vi "Write Image.vi"(0 "Session In":T1, 1 "Folder":string, 2 "Image Name":string, 3 "Camera Missing?":bool, 5 "Error In":errorcluster, 6 "Student ID":i32) -> (14 "Session Out":T1, 16 "Image Out":T2, 19 "Error Out":errorcluster)   [LabVIEW 2013]
uses:
  <vilib>/vision/Image Controls.llb/IMAQ Image.ctl
  <vilib>/userdefined/High Color/IMAQdx.ctl
  <vilib>/vision/driver/NI_Vision_Acquisition_Software.lvlib
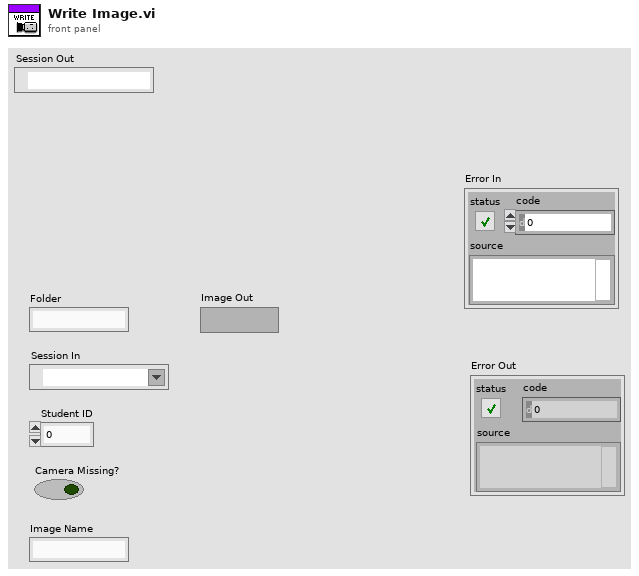
[diagram p1: front panel]
types:
  T1 = typedef "IMAQdx.ctl" = refnum<k21>
  T2 = typedef "IMAQ Image.ctl" = refnum<image>
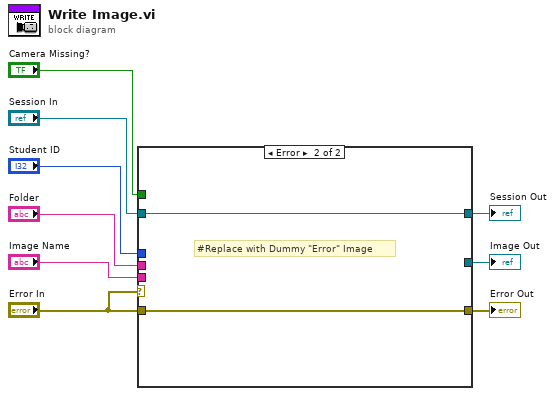
[diagram p0: block diagram]
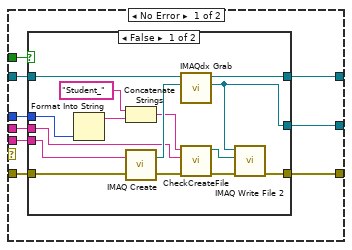
[diagram p2: hidden frame]
diagram:
  n1 = case shown="Error" "Error In" {
    tunnel: "Image Name" -> [w18 _]
    tunnel: "Folder" -> [w17 _]
    tunnel: "Student ID" -> [w16 _]
    tunnel: "Camera Missing?" -> [w15 _]
    tunnel: [w14 _] -> w5
    tunnel: "Session In" -> [w13 w36]
    tunnel: [w12 w36] -> w3
    tunnel: [w11 w37] -> w2
    tunnel: "Error In" -> [w10 w37]
    frame No Error {
      n2 = case shown="False" w15 {
        tunnel: w13 -> [w33 w35]
        tunnel: [w31 _] -> w14
        tunnel: w16 -> [w26 _]
        tunnel: w17 -> [w25 _]
        tunnel: w18 -> [w24 _]
        tunnel: [w23 w35] -> w12
        tunnel: [w21 w34] -> w11
        tunnel: w10 -> [w20 w34]
        frame False {
          n3 = Format Into String(w26) -> (resulting string=w28:string)  [unwired: 3 in, 1 out]
          n4 = Concatenate Strings("Student_" ("string"), w28) -> (w27:string)
          n5 = call "IMAQ Create"("Image Name"=w24, "error in (no error)"=w20) -> ("New Image"=w32:T2, "error out"=w19:errorcluster)  [unwired: 2 in, 1 out]
          n6 = call <vilib>:"IMAQdx Grab.vi"("Image In"=w32, "Session In"=w33) -> ("Image Out"=w31:T2, "Session Out"=w23:T1)  [unwired: 2 in, 6 out]
          n7 = call "CheckCreateFile.vi"("Error In"=w19, "Folder"=w25, "Image Name"=w27) -> ("Error Out"=w22:errorcluster, "File Path"=w30:path)  [unwired: 7 in]
          n8 = call-poly "IMAQ Write File 2"("error in (no error)"=w22, "File Path"=w30, "Image"=w31) -> ("error out"=w21:errorcluster)  [unwired: 7 in, 1 out]
        }
        frame True {
        }
      }
    }
    frame Error {
      # "#Replace with Dummy \"Error\" Image"
    }
  }
  "Image Out" <- w5
  "Session Out" <- w3
  "Error Out" <- w2
